vi "MaxEye_ATE_Create Configuration Variable to Text.vi"(0 "Variant":variant, 11 "error in (no error)":errorcluster) -> (4 "concatenated string":string, 15 "error out":errorcluster)   [LabVIEW 2021]
uses:
  <vilib>/Utility/Data Type/NI_Data Type.lvlib
  <userlib>/_OpenG.lib/lvdata/lvdata.llb/openg_variant.lvlib
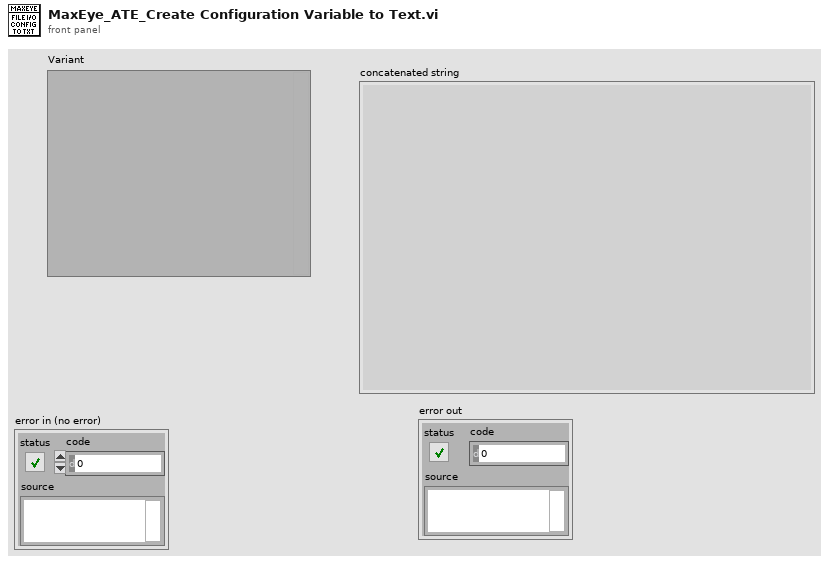
[diagram p1: front panel]
types:
  T1 = typedef "NI_Data Type.lvlib/Data Type.ctl" = enum8{"Invalid Type", "Void", "I8", "I16", "I32", "I64", "U8", "U16", "U32", "U64", "Single Float", "Double Float", "Extended Float", "Single Complex", "Double Complex", "Extended Complex", "Enum U8", "Enum U16", "Enum U32", "Enum U64", "Single Float With Unit", "Double Float With Unit", "Extended Float With Unit", "Single Complex with Unit", "Double Complex with Unit", "Extended Complex with Unit", "Boolean", "String", "Path", "Picture", "Tag", "Array", "Cluster", "Variant", "LV Variant", "Waveform", "Timestamp", "Digital Waveform", "Digital Data", "ExpressData", "Refnum", "External Data", "VI", "Poly VI", "LabVIEW Class Instance", "Fixed Point", "Set Collection", "Map Collection"}
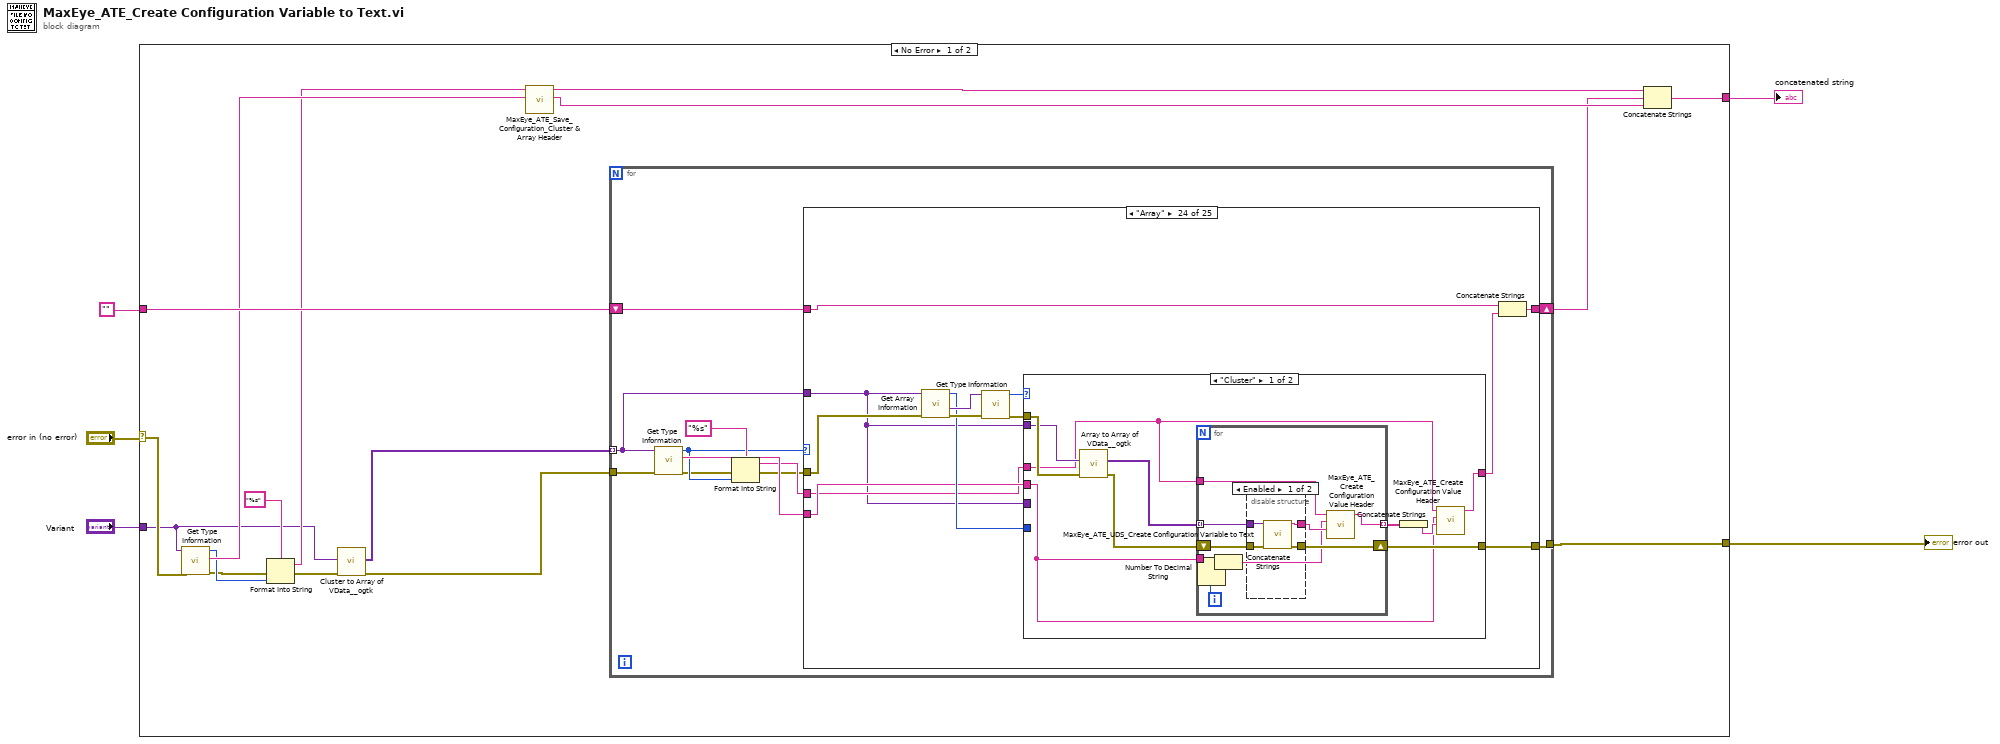
[diagram p0: block diagram]
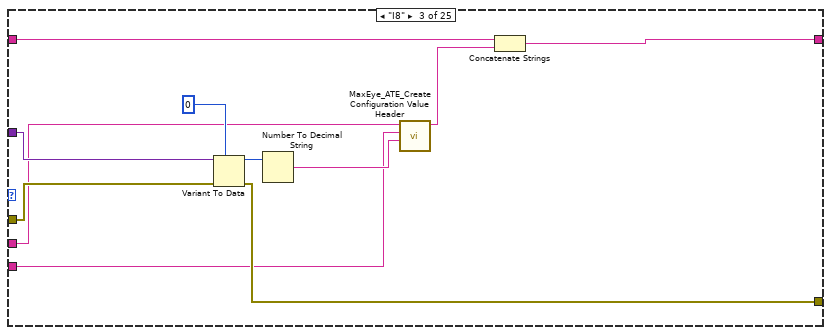
[diagram p4: hidden frame]
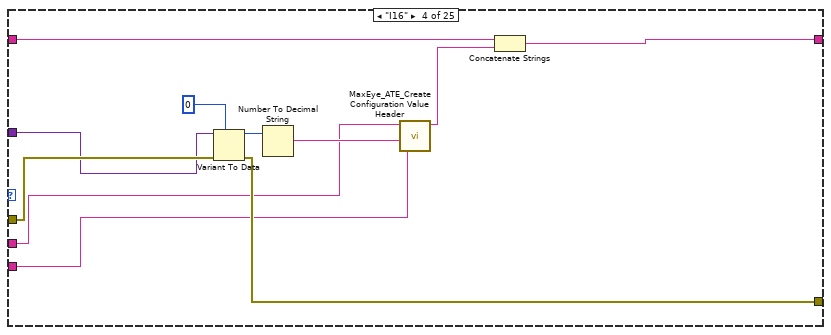
[diagram p5: hidden frame]
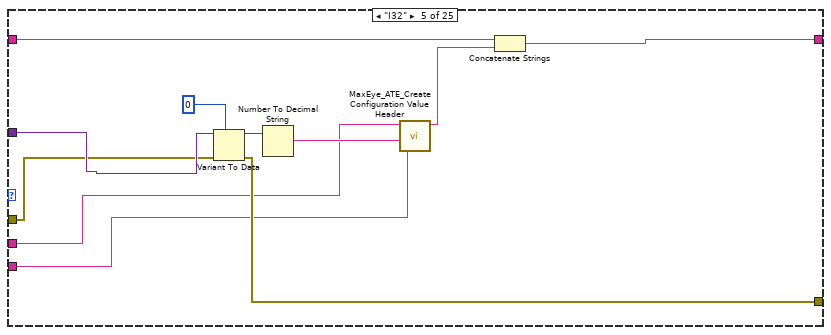
[diagram p6: hidden frame]
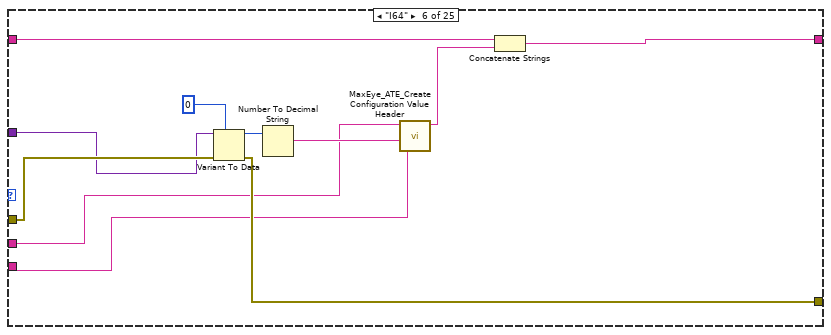
[diagram p7: hidden frame]
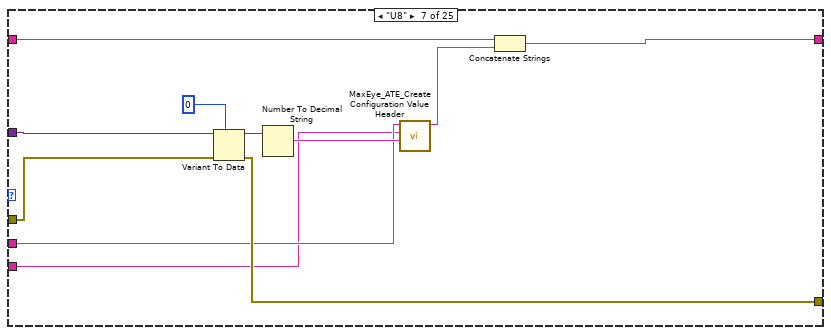
[diagram p8: hidden frame]
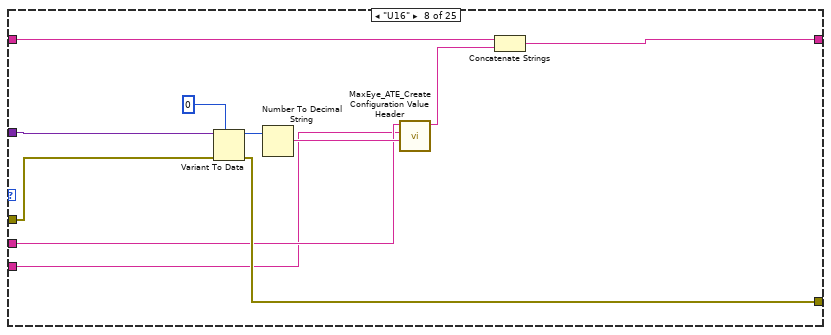
[diagram p9: hidden frame]
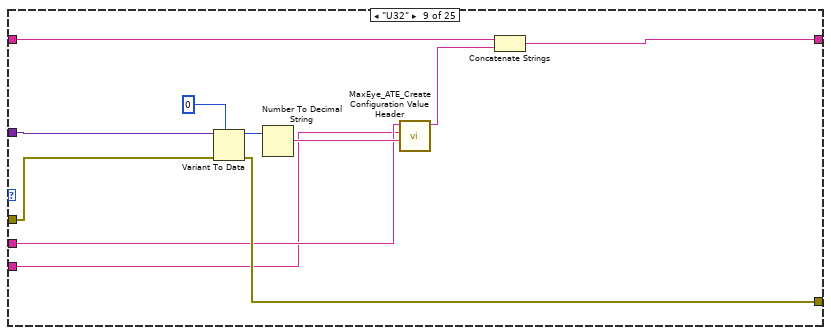
[diagram p10: hidden frame]
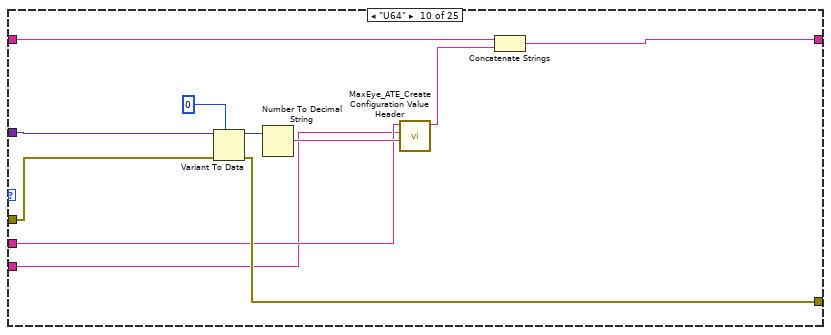
[diagram p11: hidden frame]
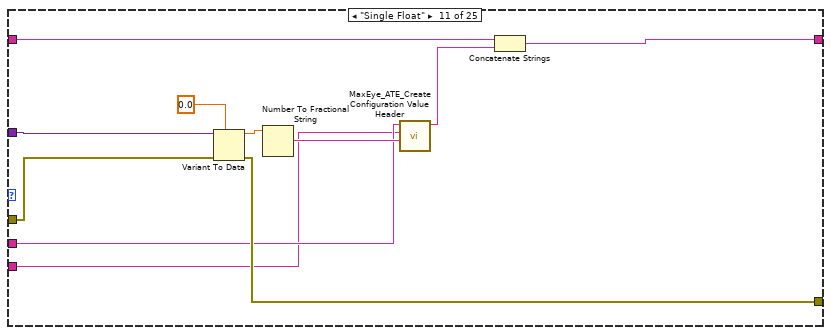
[diagram p12: hidden frame]
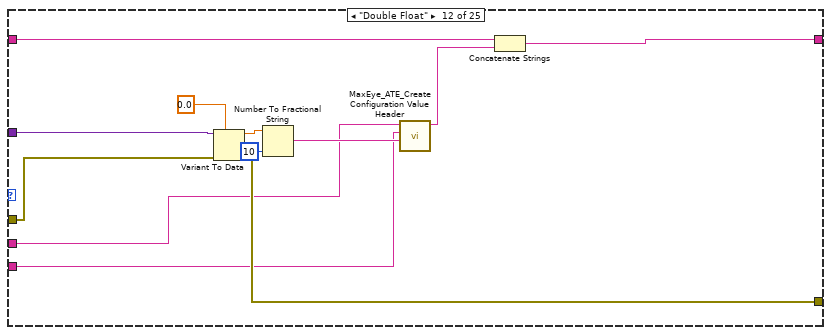
[diagram p13: hidden frame]
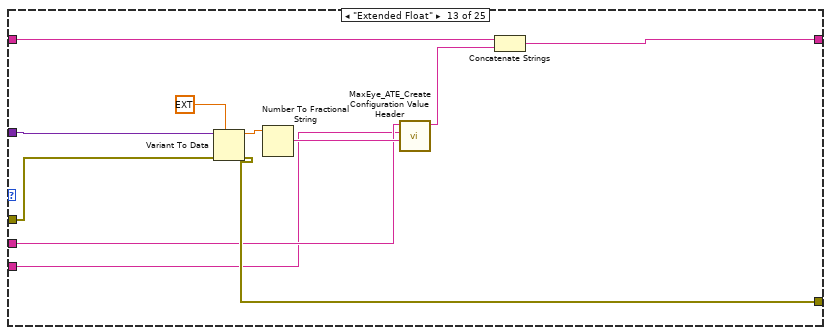
[diagram p14: hidden frame]
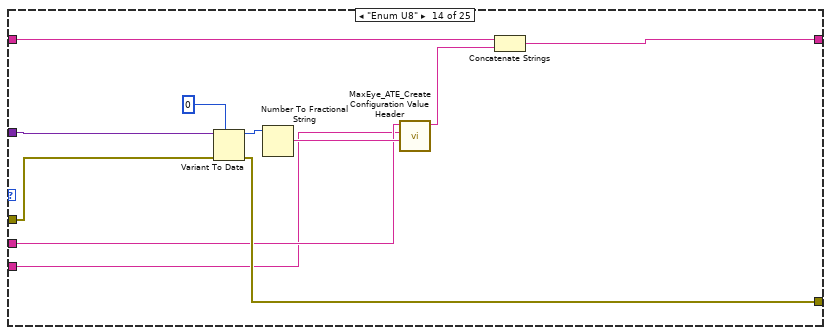
[diagram p15: hidden frame]
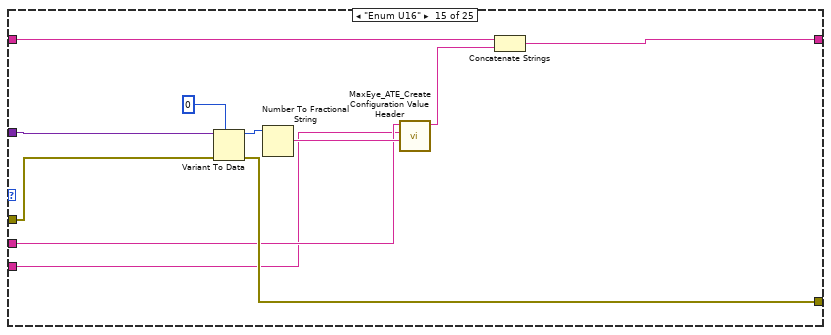
[diagram p16: hidden frame]
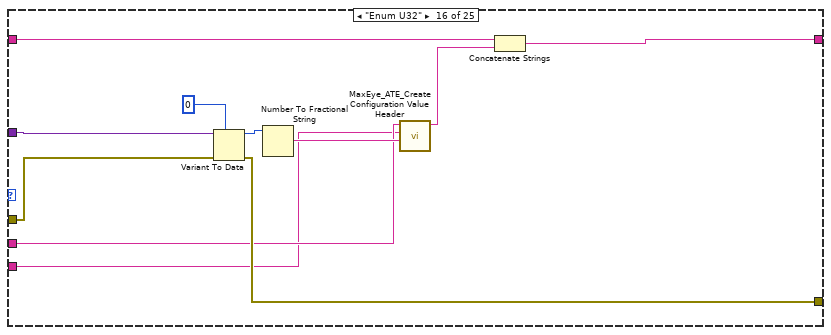
[diagram p17: hidden frame]
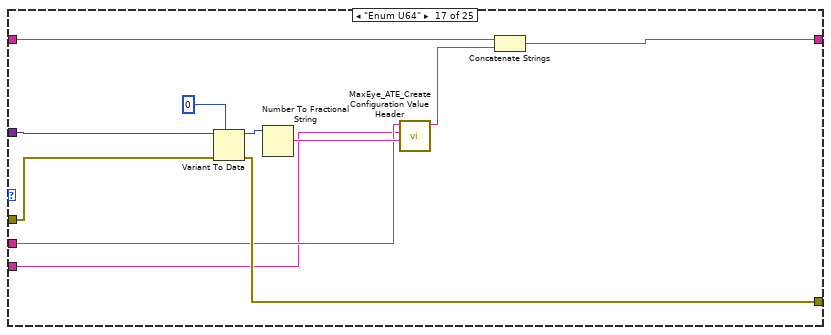
[diagram p18: hidden frame]
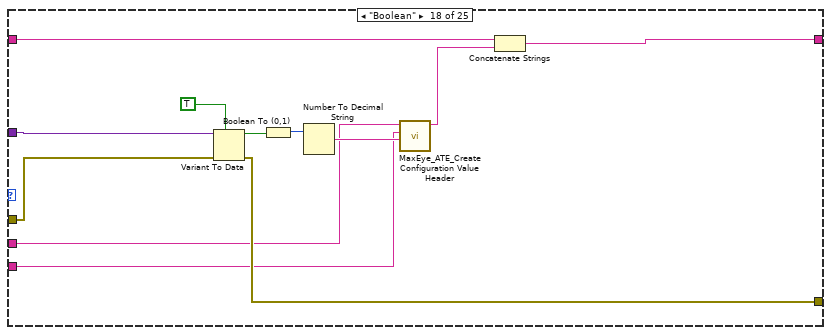
[diagram p19: hidden frame]
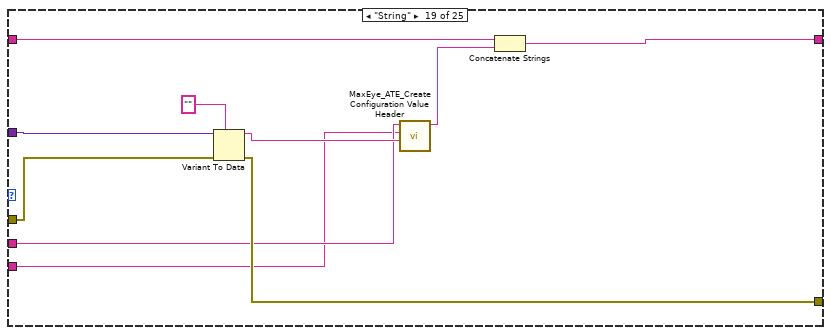
[diagram p20: hidden frame]
diagram:
  n1 = case shown="No Error" "error in (no error)" {
    selector: "error in (no error)" -> [w15 w1033]
    tunnel: "" -> [w21 w1032]
    tunnel: [w17 w1032] -> w4
    tunnel: [w16 w1033] -> w2
    tunnel: "Variant" -> [w9 _]
    frame No Error {
      n2 = call <vilib>:"Get Type Information.vi"("error in (no error)"=w15, "variant"=w9) -> ("error out"=w10:errorcluster, "name"=w14:string, "type"=w13:T1)  [unwired: 5 in, 2 out]
      n3 = Format Into String(format string="%s", error in=w10, w13) -> (resulting string=w11:string, error out=w6:errorcluster)  [unwired: 1 in]
      n4 = call <userlib>:"Cluster to Array of VData__ogtk.vi"("error in (no error)"=w6, "Cluster"=w9) -> ("error out"=w7:errorcluster, "Array of VData"=w8:variant[])  [unwired: 8 in]
      n5 = call "MaxEye_ATE_Save_Configuration_Cluster & Array Header.vi"("Label Name"=w14, "Class Name"=w11) -> ("End"=w19:string, "Begin"=w20:string)  [unwired: 8 in]
      n6 = for {
        tunnel: w7 -> [w32]
        shift-right: [w30] -> w18
        shift-left: w21 -> [w31]
        tunnel: [w29] -> w16
        tunnel: w8 -> [w22] mode=indexing
        n7 = call <vilib>:"Get Type Information.vi"("error in (no error)"=w32, "variant"=w22) -> ("error out"=w23:errorcluster, "name"=w28:string, "type"=w26:T1)  [unwired: 5 in, 2 out]
        n8 = Format Into String(format string="%s", error in=w23, w26) -> (resulting string=w25:string, error out=w24:errorcluster)  [unwired: 1 in]
        n9 = case shown="\"Array\"" w26 {
          tunnel: w24 -> [w33 w35 w47 w51 w61 w73 w91 w102 w113 w124 w135 w147 w158 w169 w180 w191 w202 w214 w224 w235 w244 w247 w264 w277 w1031]
          tunnel: w31 -> [w34 w36 w44 w56 w67 w78 w88 w99 w110 w121 w132 w144 w155 w166 w177 w188 w199 w212 w222 w233 w243 w255 w263 w276 w1030]
          tunnel: [w34 w36 w43 w55 w66 w77 w87 w98 w109 w120 w131 w143 w154 w165 w176 w187 w198 w211 w221 w232 w242 w254 w262 w275 w1029] -> w30
          tunnel: [w33 w35 w40 w52 w63 w74 w84 w95 w106 w117 w128 w140 w151 w162 w173 w184 w195 w206 w218 w228 w244 w247 w264 w268 w1028] -> w29
          tunnel: w28 -> [_ _ w37 w49 w59 w70 w81 w92 w103 w114 w125 w139 w148 w159 w170 w181 w192 w203 w215 w225 w239 w251 w259 w267 _]
          tunnel: w25 -> [_ _ w38 w50 w60 w71 w82 w93 w104 w115 w126 w138 w149 w160 w171 w182 w193 w204 w216 w226 w240 w252 w260 w266 _]
          tunnel: w22 -> [_ _ w39 w48 w62 w72 w83 w94 w105 w116 w127 w137 w150 w161 w172 w183 w194 w205 w217 w227 w238 w250 w258 w265 w1026]
          frame "Invalid Type", Default {
          }
          frame "Void" {
          }
          frame "I8" {
            n10 = Variant To Data(error in=w47, type=i8 0, Variant=w39) -> (data=w45:i8, error out=w40:errorcluster)
            n11 = Number To Decimal String(number=w45) -> (decimal integer string=w42:string)  [unwired: 1 in]
            n12 = call "MaxEye_ATE_Create Configuration Value Header.vi"("Class_value"=w42, "Label_name"=w37, "Class_name"=w38) -> ("Encoded Value"=w41:string)  [unwired: 8 in]
            n13 = Concatenate Strings(w44, w41) -> (w43:string)
          }
          frame "I16" {
            n14 = Variant To Data(error in=w51, type=i16 0, Variant=w48) -> (data=w57:i16, error out=w52:errorcluster)
            n15 = Number To Decimal String(number=w57) -> (decimal integer string=w54:string)  [unwired: 1 in]
            n16 = call "MaxEye_ATE_Create Configuration Value Header.vi"("Class_value"=w54, "Label_name"=w49, "Class_name"=w50) -> ("Encoded Value"=w53:string)  [unwired: 8 in]
            n17 = Concatenate Strings(w56, w53) -> (w55:string)
          }
          frame "I32" {
            n18 = Variant To Data(error in=w61, type=0, Variant=w62) -> (data=w68:i32, error out=w63:errorcluster)
            n19 = Number To Decimal String(number=w68) -> (decimal integer string=w65:string)  [unwired: 1 in]
            n20 = call "MaxEye_ATE_Create Configuration Value Header.vi"("Class_value"=w65, "Label_name"=w59, "Class_name"=w60) -> ("Encoded Value"=w64:string)  [unwired: 8 in]
            n21 = Concatenate Strings(w67, w64) -> (w66:string)
          }
          frame "I64" {
            n22 = Variant To Data(error in=w73, type=i64 0, Variant=w72) -> (data=w79:i64, error out=w74:errorcluster)
            n23 = Number To Decimal String(number=w79) -> (decimal integer string=w76:string)  [unwired: 1 in]
            n24 = call "MaxEye_ATE_Create Configuration Value Header.vi"("Class_value"=w76, "Label_name"=w70, "Class_name"=w71) -> ("Encoded Value"=w75:string)  [unwired: 8 in]
            n25 = Concatenate Strings(w78, w75) -> (w77:string)
          }
          frame "U8" {
            n26 = Variant To Data(error in=w91, type=u8 0, Variant=w83) -> (data=w89:u8, error out=w84:errorcluster)
            n27 = Number To Decimal String(number=w89) -> (decimal integer string=w86:string)  [unwired: 1 in]
            n28 = call "MaxEye_ATE_Create Configuration Value Header.vi"("Class_value"=w86, "Label_name"=w81, "Class_name"=w82) -> ("Encoded Value"=w85:string)  [unwired: 8 in]
            n29 = Concatenate Strings(w88, w85) -> (w87:string)
          }
          frame "U16" {
            n30 = Variant To Data(error in=w102, type=u16 0, Variant=w94) -> (data=w100:u16, error out=w95:errorcluster)
            n31 = Number To Decimal String(number=w100) -> (decimal integer string=w97:string)  [unwired: 1 in]
            n32 = call "MaxEye_ATE_Create Configuration Value Header.vi"("Class_value"=w97, "Label_name"=w92, "Class_name"=w93) -> ("Encoded Value"=w96:string)  [unwired: 8 in]
            n33 = Concatenate Strings(w99, w96) -> (w98:string)
          }
          frame "U32" {
            n34 = Variant To Data(error in=w113, type=u32 0, Variant=w105) -> (data=w111:u32, error out=w106:errorcluster)
            n35 = Number To Decimal String(number=w111) -> (decimal integer string=w108:string)  [unwired: 1 in]
            n36 = call "MaxEye_ATE_Create Configuration Value Header.vi"("Class_value"=w108, "Label_name"=w103, "Class_name"=w104) -> ("Encoded Value"=w107:string)  [unwired: 8 in]
            n37 = Concatenate Strings(w110, w107) -> (w109:string)
          }
          frame "U64" {
            n38 = Variant To Data(error in=w124, type=u64 0, Variant=w116) -> (data=w122:u64, error out=w117:errorcluster)
            n39 = Number To Decimal String(number=w122) -> (decimal integer string=w119:string)  [unwired: 1 in]
            n40 = call "MaxEye_ATE_Create Configuration Value Header.vi"("Class_value"=w119, "Label_name"=w114, "Class_name"=w115) -> ("Encoded Value"=w118:string)  [unwired: 8 in]
            n41 = Concatenate Strings(w121, w118) -> (w120:string)
          }
          frame "Single Float" {
            n42 = Variant To Data(error in=w135, type=sgl 0.0, Variant=w127) -> (data=w133:sgl, error out=w128:errorcluster)
            n43 = Number To Fractional String(number=w133) -> (F-format string=w130:string)  [unwired: 3 in]
            n44 = call "MaxEye_ATE_Create Configuration Value Header.vi"("Class_value"=w130, "Label_name"=w125, "Class_name"=w126) -> ("Encoded Value"=w129:string)  [unwired: 8 in]
            n45 = Concatenate Strings(w132, w129) -> (w131:string)
          }
          frame "Double Float" {
            n46 = Variant To Data(error in=w147, type=0.0, Variant=w137) -> (data=w145:dbl, error out=w140:errorcluster)
            n47 = Number To Fractional String(number=w145, precision (6)=i16 10) -> (F-format string=w142:string)  [unwired: 2 in]
            n48 = call "MaxEye_ATE_Create Configuration Value Header.vi"("Class_value"=w142, "Label_name"=w139, "Class_name"=w138) -> ("Encoded Value"=w141:string)  [unwired: 8 in]
            n49 = Concatenate Strings(w144, w141) -> (w143:string)
          }
          frame "Extended Float" {
            n50 = Variant To Data(error in=w158, type=ext 0.0, Variant=w150) -> (data=w156:ext, error out=w151:errorcluster)
            n51 = Number To Fractional String(number=w156) -> (F-format string=w153:string)  [unwired: 3 in]
            n52 = call "MaxEye_ATE_Create Configuration Value Header.vi"("Class_value"=w153, "Label_name"=w148, "Class_name"=w149) -> ("Encoded Value"=w152:string)  [unwired: 8 in]
            n53 = Concatenate Strings(w155, w152) -> (w154:string)
          }
          frame "Enum U8" {
            n54 = Variant To Data(error in=w169, type=u8 0, Variant=w161) -> (data=w167:u8, error out=w162:errorcluster)
            n55 = Number To Fractional String(number=w167) -> (F-format string=w164:string)  [unwired: 3 in]
            n56 = call "MaxEye_ATE_Create Configuration Value Header.vi"("Class_value"=w164, "Label_name"=w159, "Class_name"=w160) -> ("Encoded Value"=w163:string)  [unwired: 8 in]
            n57 = Concatenate Strings(w166, w163) -> (w165:string)
          }
          frame "Enum U16" {
            n58 = Variant To Data(error in=w180, type=u16 0, Variant=w172) -> (data=w178:u16, error out=w173:errorcluster)
            n59 = Number To Fractional String(number=w178) -> (F-format string=w175:string)  [unwired: 3 in]
            n60 = call "MaxEye_ATE_Create Configuration Value Header.vi"("Class_value"=w175, "Label_name"=w170, "Class_name"=w171) -> ("Encoded Value"=w174:string)  [unwired: 8 in]
            n61 = Concatenate Strings(w177, w174) -> (w176:string)
          }
          frame "Enum U32" {
            n62 = Variant To Data(error in=w191, type=u32 0, Variant=w183) -> (data=w189:u32, error out=w184:errorcluster)
            n63 = Number To Fractional String(number=w189) -> (F-format string=w186:string)  [unwired: 3 in]
            n64 = call "MaxEye_ATE_Create Configuration Value Header.vi"("Class_value"=w186, "Label_name"=w181, "Class_name"=w182) -> ("Encoded Value"=w185:string)  [unwired: 8 in]
            n65 = Concatenate Strings(w188, w185) -> (w187:string)
          }
          frame "Enum U64" {
            n66 = Variant To Data(error in=w202, type=u64 0, Variant=w194) -> (data=w200:u64, error out=w195:errorcluster)
            n67 = Number To Fractional String(number=w200) -> (F-format string=w197:string)  [unwired: 3 in]
            n68 = call "MaxEye_ATE_Create Configuration Value Header.vi"("Class_value"=w197, "Label_name"=w192, "Class_name"=w193) -> ("Encoded Value"=w196:string)  [unwired: 8 in]
            n69 = Concatenate Strings(w199, w196) -> (w198:string)
          }
          frame "Boolean" {
            n70 = Variant To Data(error in=w214, type=TRUE, Variant=w205) -> (data=w209:bool, error out=w206:errorcluster)
            n71 = Boolean To (0,1)(Boolean=w209) -> (0, 1=w208:i16)
            n72 = Number To Decimal String(number=w208) -> (decimal integer string=w207:string)  [unwired: 1 in]
            n73 = call "MaxEye_ATE_Create Configuration Value Header.vi"("Class_value"=w207, "Label_name"=w203, "Class_name"=w204) -> ("Encoded Value"=w210:string)  [unwired: 8 in]
            n74 = Concatenate Strings(w212, w210) -> (w211:string)
          }
          frame "String" {
            n75 = Variant To Data(error in=w224, type="", Variant=w217) -> (data=w219:string, error out=w218:errorcluster)
            n76 = call "MaxEye_ATE_Create Configuration Value Header.vi"("Class_value"=w219, "Label_name"=w215, "Class_name"=w216) -> ("Encoded Value"=w220:string)  [unwired: 8 in]
            n77 = Concatenate Strings(w222, w220) -> (w221:string)
          }
          frame "Path" {
            n78 = Variant To Data(error in=w235, type=path "", Variant=w227) -> (data=w230:path, error out=w228:errorcluster)
            n79 = Path To String(path=w230) -> (string=w229:string)
            n80 = call "MaxEye_ATE_Create Configuration Value Header.vi"("Class_value"=w229, "Label_name"=w225, "Class_name"=w226) -> ("Encoded Value"=w231:string)  [unwired: 8 in]
            n81 = Concatenate Strings(w233, w231) -> (w232:string)
          }
          frame "Refnum" {
            n82 = Variant To Data(type="", Variant=w238) -> (data=w236:string)  [unwired: 1 in, 1 out]
            n83 = call "MaxEye_ATE_Create Configuration Value Header.vi"("Class_value"=w236, "Label_name"=w239, "Class_name"=w240) -> ("Encoded Value"=w241:string)  [unwired: 8 in]
            n84 = Concatenate Strings(w243, w241) -> (w242:string)
          }
          frame "Timestamp" {
            n85 = Variant To Data(error in=w247, type=timestamp(0 s since 1904-01-01), Variant=w250) -> (data=w246:timestamp)  [unwired: 1 out]
            n86 = To Double Precision Float(number=w246) -> (double precision float=w245:dbl)
            n87 = Number To Fractional String(number=w245) -> (F-format string=w248:string)  [unwired: 3 in]
            n88 = call "MaxEye_ATE_Create Configuration Value Header.vi"("Class_value"=w248, "Label_name"=w251, "Class_name"=w252) -> ("Encoded Value"=w253:string)  [unwired: 8 in]
            n89 = Concatenate Strings(w255, w253) -> (w254:string)
          }
          frame "Tag" {
            n90 = Variant To Data(type="", Variant=w258) -> (data=w256:string)  [unwired: 1 in, 1 out]
            n91 = call "MaxEye_ATE_Create Configuration Value Header.vi"("Class_value"=w256, "Label_name"=w259, "Class_name"=w260) -> ("Encoded Value"=w261:string)  [unwired: 8 in]
            n92 = Concatenate Strings(w263, w261) -> (w262:string)
          }
          frame "Array" {
            n93 = call <vilib>:"Get Array Information.vi"("error in (no error)"=w277, "variant"=w265) -> ("error out"=w273:errorcluster, "array element data type"=w274:variant, "number of dimensions"=w272:i32)  [unwired: 6 in, 1 out]
            n94 = call <vilib>:"Get Type Information.vi"("error in (no error)"=w273, "variant"=w274) -> ("error out"=w270:errorcluster, "type"=w271:T1)  [unwired: 5 in, 3 out]
            n95 = case shown="\"Cluster\"" w271 {
              selector: w271 -> [_ w308]
              tunnel: w272 -> [_ w309]
              tunnel: w270 -> [w287 w304]
              tunnel: w266 -> [w279 w307]
              tunnel: w267 -> [w278 w306]
              tunnel: w265 -> [_ w305]
              tunnel: [w281 w303] -> w269
              tunnel: [w283 w302] -> w268
              tunnel: w265 -> [w286 _]
              frame "Cluster" {
                n96 = call <userlib>:"Array to Array of VData__ogtk.vi"("error in (no error)"=w287, "MultiD Array"=w286) -> ("error out"=w284:errorcluster, "1D Array of Variants"=w285:variant[])  [unwired: 8 in]
                n97 = for {
                  tunnel: w285 -> [w297] mode=indexing
                  tunnel: [w293] -> w282 mode=indexing
                  shift-right: [w295] -> w283
                  shift-left: w284 -> [w296]
                  tunnel: w279 -> [w292]
                  tunnel: w278 -> [w291]
                  i -> [w290]
                  n98 = Number To Decimal String(number=w290) -> (decimal integer string=w289:string)  [unwired: 1 in]
                  n99 = Concatenate Strings(w291, w289) -> (w288:string)
                  n100 = disable-structure shown="Enabled" {
                    disable-tunnel: w297 -> [w298 _]
                    disable-tunnel: w296 -> [w301 _]
                    disable-tunnel: [w300 _] -> w295
                    disable-tunnel: [w299 _] -> w294
                    frame Enabled {
                      n101 = call "MaxEye_ATE_UDS_Create Configuration Variable to Text.vi"("Variant"=w298, "error in (no error)"=w301) -> ("concatenated string"=w299:string, "error out"=w300:errorcluster)  [unwired: 12 in]
                    }
                    frame Disabled {
                    }
                  }
                  n102 = call "MaxEye_ATE_Create Configuration Value Header.vi"("Class_value"=w294, "Label_name"=w288, "Class_name"=w292) -> ("Encoded Value"=w293:string)  [unwired: 8 in]
                }
                n103 = Concatenate Strings(w282) -> (w280:string)
                n104 = call "MaxEye_ATE_Create Configuration Value Header.vi"("Class_value"=w280, "Label_name"=w278, "Class_name"=w279) -> ("Encoded Value"=w281:string)  [unwired: 8 in]
              }
              frame "Void", Default {
                n105 = case shown="1" w309 {
                  tunnel: w308 -> [_ w317 w574 w803]
                  tunnel: w307 -> [_ w316 w573 w802]
                  tunnel: w306 -> [_ w315 w572 w801]
                  tunnel: w305 -> [_ w314 w571 w800]
                  tunnel: w304 -> [w310 w313 w570 w799]
                  tunnel: [_ w312 w569 w798] -> w303
                  tunnel: [w310 w311 w568 w797] -> w302
                  frame 0, Default {
                  }
                  frame 1 {
                    n106 = case shown="\"Enum U32\"" w317 {
                      tunnel: w316 -> [w328 w339 w350 w361 w372 w383 w394 w405 w416 w427 w438 w449 w460 w473 w484 w495 w506 w517 w528 w539 w551 w566 _]
                      tunnel: w315 -> [w327 w338 w349 w360 w371 w382 w393 w404 w415 w426 w437 w448 w459 w472 w483 w494 w505 w516 w527 w538 w550 w565 _]
                      tunnel: w314 -> [w325 w336 w347 w358 w369 w380 w391 w402 w413 w424 w435 w446 w457 w464 w481 w492 w503 w514 w525 w536 w548 w563 _]
                      tunnel: w313 -> [w326 w337 w348 w359 w370 w381 w392 w403 w414 w425 w436 w447 w458 w463 w482 w493 w504 w515 w526 w537 w549 w564 w567]
                      tunnel: [w319 w330 w341 w352 w363 w374 w385 w396 w407 w418 w429 w440 w451 w468 w475 w486 w497 w508 w519 w530 w543 w557 _] -> w312
                      tunnel: [w318 w329 w340 w351 w362 w373 w384 w395 w406 w417 w428 w439 w450 w462 w474 w485 w496 w507 w518 w529 w542 w555 w567] -> w311
                      frame "I8" {
                        n107 = Variant To Data(error in=w326, type=i8[] [], Variant=w325) -> (data=w323:i8[], error out=w318:errorcluster)
                        n108 = Array To Spreadsheet String(delimiter (Tab)=",", array=w323, 3:"%s" ("format string")) -> (spreadsheet string=w320:string)
                        n109 = call "MaxEye_ATE_Create Configuration Value Header.vi"("Class_value"=w320, "Label_name"=w327, "Class_name"=w328) -> ("Encoded Value"=w319:string)  [unwired: 8 in]
                      }
                      frame "I16" {
                        n110 = Variant To Data(error in=w337, type=i16[] [], Variant=w336) -> (data=w334:i16[], error out=w329:errorcluster)
                        n111 = Array To Spreadsheet String(delimiter (Tab)=",", array=w334, 3:"%s" ("format string")) -> (spreadsheet string=w331:string)
                        n112 = call "MaxEye_ATE_Create Configuration Value Header.vi"("Class_value"=w331, "Label_name"=w338, "Class_name"=w339) -> ("Encoded Value"=w330:string)  [unwired: 8 in]
                      }
                      frame "I32" {
                        n113 = Variant To Data(error in=w348, type=i32[] [], Variant=w347) -> (data=w345:i32[], error out=w340:errorcluster)
                        n114 = Array To Spreadsheet String(delimiter (Tab)=",", array=w345, 3:"%s" ("format string")) -> (spreadsheet string=w342:string)
                        n115 = call "MaxEye_ATE_Create Configuration Value Header.vi"("Class_value"=w342, "Label_name"=w349, "Class_name"=w350) -> ("Encoded Value"=w341:string)  [unwired: 8 in]
                      }
                      frame "I64" {
                        n116 = Variant To Data(error in=w359, type=i64[] [], Variant=w358) -> (data=w356:i64[], error out=w351:errorcluster)
                        n117 = Array To Spreadsheet String(delimiter (Tab)=",", array=w356, 3:"%s" ("format string")) -> (spreadsheet string=w353:string)
                        n118 = call "MaxEye_ATE_Create Configuration Value Header.vi"("Class_value"=w353, "Label_name"=w360, "Class_name"=w361) -> ("Encoded Value"=w352:string)  [unwired: 8 in]
                      }
                      frame "U8" {
                        n119 = Variant To Data(error in=w370, type=u8[] [], Variant=w369) -> (data=w367:u8[], error out=w362:errorcluster)
                        n120 = Array To Spreadsheet String(delimiter (Tab)=",", array=w367, 3:"%s" ("format string")) -> (spreadsheet string=w364:string)
                        n121 = call "MaxEye_ATE_Create Configuration Value Header.vi"("Class_value"=w364, "Label_name"=w371, "Class_name"=w372) -> ("Encoded Value"=w363:string)  [unwired: 8 in]
                      }
                      frame "U16" {
                        n122 = Variant To Data(error in=w381, type=u16[] [], Variant=w380) -> (data=w378:u16[], error out=w373:errorcluster)
                        n123 = Array To Spreadsheet String(delimiter (Tab)=",", array=w378, 3:"%s" ("format string")) -> (spreadsheet string=w375:string)
                        n124 = call "MaxEye_ATE_Create Configuration Value Header.vi"("Class_value"=w375, "Label_name"=w382, "Class_name"=w383) -> ("Encoded Value"=w374:string)  [unwired: 8 in]
                      }
                      frame "U32" {
                        n125 = Variant To Data(error in=w392, type=u32[] [], Variant=w391) -> (data=w389:u32[], error out=w384:errorcluster)
                        n126 = Array To Spreadsheet String(delimiter (Tab)=",", array=w389, 3:"%s" ("format string")) -> (spreadsheet string=w386:string)
                        n127 = call "MaxEye_ATE_Create Configuration Value Header.vi"("Class_value"=w386, "Label_name"=w393, "Class_name"=w394) -> ("Encoded Value"=w385:string)  [unwired: 8 in]
                      }
                      frame "U64" {
                        n128 = Variant To Data(error in=w403, type=u64[] [], Variant=w402) -> (data=w400:u64[], error out=w395:errorcluster)
                        n129 = Array To Spreadsheet String(delimiter (Tab)=",", array=w400, 3:"%s" ("format string")) -> (spreadsheet string=w397:string)
                        n130 = call "MaxEye_ATE_Create Configuration Value Header.vi"("Class_value"=w397, "Label_name"=w404, "Class_name"=w405) -> ("Encoded Value"=w396:string)  [unwired: 8 in]
                      }
                      frame "Single Float" {
                        n131 = Variant To Data(error in=w414, type=sgl[] [], Variant=w413) -> (data=w411:sgl[], error out=w406:errorcluster)
                        n132 = Array To Spreadsheet String(delimiter (Tab)=",", array=w411, 3:"%s" ("format string")) -> (spreadsheet string=w408:string)
                        n133 = call "MaxEye_ATE_Create Configuration Value Header.vi"("Class_value"=w408, "Label_name"=w415, "Class_name"=w416) -> ("Encoded Value"=w407:string)  [unwired: 8 in]
                      }
                      frame "Double Float" {
                        n134 = Variant To Data(error in=w425, type=dbl[] [], Variant=w424) -> (data=w422:dbl[], error out=w417:errorcluster)
                        n135 = Array To Spreadsheet String(delimiter (Tab)=",", array=w422, 3:"%s" ("format string")) -> (spreadsheet string=w419:string)
                        n136 = call "MaxEye_ATE_Create Configuration Value Header.vi"("Class_value"=w419, "Label_name"=w426, "Class_name"=w427) -> ("Encoded Value"=w418:string)  [unwired: 8 in]
                      }
                      frame "Extended Float" {
                        n137 = Variant To Data(error in=w436, type=ext[] [], Variant=w435) -> (data=w433:ext[], error out=w428:errorcluster)
                        n138 = Array To Spreadsheet String(delimiter (Tab)=",", array=w433, 3:"%s" ("format string")) -> (spreadsheet string=w430:string)
                        n139 = call "MaxEye_ATE_Create Configuration Value Header.vi"("Class_value"=w430, "Label_name"=w437, "Class_name"=w438) -> ("Encoded Value"=w429:string)  [unwired: 8 in]
                      }
                      frame "Single Complex" {
                        n140 = Variant To Data(error in=w447, type=ext[] [], Variant=w446) -> (data=w444:ext[], error out=w439:errorcluster)
                        n141 = Array To Spreadsheet String(delimiter (Tab)=",", array=w444, 3:"%s" ("format string")) -> (spreadsheet string=w441:string)
                        n142 = call "MaxEye_ATE_Create Configuration Value Header.vi"("Class_value"=w441, "Label_name"=w448, "Class_name"=w449) -> ("Encoded Value"=w440:string)  [unwired: 8 in]
                      }
                      frame "Double Complex" {
                        n143 = Variant To Data(error in=w458, type=ext[] [], Variant=w457) -> (data=w455:ext[], error out=w450:errorcluster)
                        n144 = Array To Spreadsheet String(delimiter (Tab)=",", array=w455, 3:"%s" ("format string")) -> (spreadsheet string=w452:string)
                        n145 = call "MaxEye_ATE_Create Configuration Value Header.vi"("Class_value"=w452, "Label_name"=w459, "Class_name"=w460) -> ("Encoded Value"=w451:string)  [unwired: 8 in]
                      }
                      frame "Timestamp" {
                        n146 = Variant To Data(error in=w463, type=timestamp[] [], Variant=w464) -> (data=w466:timestamp[], error out=w462:errorcluster)
                        n147 = To Double Precision Float(number=w466) -> (double precision float=w467:dbl[])
                        n148 = Number To Fractional String(number=w467) -> (F-format string=w461:string[])  [unwired: 3 in]
                        n149 = Array To Spreadsheet String(delimiter (Tab)=",", array=w461, 3:"%s" ("format string")) -> (spreadsheet string=w469:string)
                        n150 = call "MaxEye_ATE_Create Configuration Value Header.vi"("Class_value"=w469, "Label_name"=w472, "Class_name"=w473) -> ("Encoded Value"=w468:string)  [unwired: 8 in]
                      }
                      frame "Extended Complex" {
                        n151 = Variant To Data(error in=w482, type=ext[] [], Variant=w481) -> (data=w479:ext[], error out=w474:errorcluster)
                        n152 = Array To Spreadsheet String(delimiter (Tab)=",", array=w479, 3:"%s" ("format string")) -> (spreadsheet string=w476:string)
                        n153 = call "MaxEye_ATE_Create Configuration Value Header.vi"("Class_value"=w476, "Label_name"=w483, "Class_name"=w484) -> ("Encoded Value"=w475:string)  [unwired: 8 in]
                      }
                      frame "Enum U8" {
                        n154 = Variant To Data(error in=w493, type=u8[] [], Variant=w492) -> (data=w490:u8[], error out=w485:errorcluster)
                        n155 = Array To Spreadsheet String(delimiter (Tab)=",", array=w490, 3:"%s" ("format string")) -> (spreadsheet string=w487:string)
                        n156 = call "MaxEye_ATE_Create Configuration Value Header.vi"("Class_value"=w487, "Label_name"=w494, "Class_name"=w495) -> ("Encoded Value"=w486:string)  [unwired: 8 in]
                      }
                      frame "Enum U16" {
                        n157 = Variant To Data(error in=w504, type=u16[] [], Variant=w503) -> (data=w501:u16[], error out=w496:errorcluster)
                        n158 = Array To Spreadsheet String(delimiter (Tab)=",", array=w501, 3:"%s" ("format string")) -> (spreadsheet string=w498:string)
                        n159 = call "MaxEye_ATE_Create Configuration Value Header.vi"("Class_value"=w498, "Label_name"=w505, "Class_name"=w506) -> ("Encoded Value"=w497:string)  [unwired: 8 in]
                      }
                      frame "Enum U32" {
                        n160 = Variant To Data(error in=w515, type=u32[] [], Variant=w514) -> (data=w512:u32[], error out=w507:errorcluster)
                        n161 = Array To Spreadsheet String(delimiter (Tab)=",", array=w512, 3:"%s" ("format string")) -> (spreadsheet string=w509:string)
                        n162 = call "MaxEye_ATE_Create Configuration Value Header.vi"("Class_value"=w509, "Label_name"=w516, "Class_name"=w517) -> ("Encoded Value"=w508:string)  [unwired: 8 in]
                      }
                      frame "Enum U64" {
                        n163 = Variant To Data(error in=w526, type=u64[] [], Variant=w525) -> (data=w523:u64[], error out=w518:errorcluster)
                        n164 = Array To Spreadsheet String(delimiter (Tab)=",", array=w523, 3:"%s" ("format string")) -> (spreadsheet string=w520:string)
                        n165 = call "MaxEye_ATE_Create Configuration Value Header.vi"("Class_value"=w520, "Label_name"=w527, "Class_name"=w528) -> ("Encoded Value"=w519:string)  [unwired: 8 in]
                      }
                      frame "String" {
                        n166 = Variant To Data(error in=w537, type=string[] [], Variant=w536) -> (data=w534:string[], error out=w529:errorcluster)
                        n167 = Array To Spreadsheet String(delimiter (Tab)=",", array=w534, 3:"%s" ("format string")) -> (spreadsheet string=w531:string)
                        n168 = call "MaxEye_ATE_Create Configuration Value Header.vi"("Class_value"=w531, "Label_name"=w538, "Class_name"=w539) -> ("Encoded Value"=w530:string)  [unwired: 8 in]
                      }
                      frame "Refnum" {
                        n169 = Variant To Data(error in=w549, type=refnum<k21>[] [""], Variant=w548) -> (data=w541:refnum<k21>[], error out=w542:errorcluster)
                        n170 = for {
                          tunnel: w541 -> [w553] mode=indexing
                          tunnel: [w554] -> w540 mode=indexing
                          n171 = Variant To Data(type="", Variant=w553) -> (data=w554:string)  [unwired: 1 in, 1 out]
                        }
                        n172 = Array To Spreadsheet String(delimiter (Tab)=",", array=w540, 3:"%s" ("format string")) -> (spreadsheet string=w544:string)
                        n173 = call "MaxEye_ATE_Create Configuration Value Header.vi"("Class_value"=w544, "Label_name"=w550, "Class_name"=w551) -> ("Encoded Value"=w543:string)  [unwired: 8 in]
                      }
                      frame "Boolean" {
                        n174 = Variant To Data(error in=w564, type=bool[] [], Variant=w563) -> (data=w561:bool[], error out=w555:errorcluster)
                        n175 = Boolean To (0,1)(Boolean=w561) -> (0, 1=w556:i16[])
                        n176 = Array To Spreadsheet String(delimiter (Tab)=",", array=w556, 3:"%s" ("format string")) -> (spreadsheet string=w558:string)
                        n177 = call "MaxEye_ATE_Create Configuration Value Header.vi"("Class_value"=w558, "Label_name"=w565, "Class_name"=w566) -> ("Encoded Value"=w557:string)  [unwired: 8 in]
                      }
                      frame "Void", Default {
                      }
                    }
                  }
                  frame 2 {
                    n178 = case shown="\"Double Complex\"" w574 {
                      tunnel: w573 -> [w585 w596 w607 w618 w629 w640 w651 w662 w673 w684 w695 w706 w717 w728 w739 w750 w761 w772 w783 w795 _]
                      tunnel: w572 -> [w584 w595 w606 w617 w628 w639 w650 w661 w672 w683 w694 w705 w716 w727 w738 w749 w760 w771 w782 w794 _]
                      tunnel: w571 -> [w582 w593 w604 w615 w626 w637 w648 w659 w670 w681 w692 w703 w714 w725 w736 w747 w758 w769 w780 w792 _]
                      tunnel: w570 -> [w583 w594 w605 w616 w627 w638 w649 w660 w671 w682 w693 w704 w715 w726 w737 w748 w759 w770 w781 w793 w796]
                      tunnel: [w576 w587 w598 w609 w620 w631 w642 w653 w664 w675 w686 w697 w708 w719 w730 w741 w752 w763 w774 w786 _] -> w569
                      tunnel: [w575 w586 w597 w608 w619 w630 w641 w652 w663 w674 w685 w696 w707 w718 w729 w740 w751 w762 w773 w784 w796] -> w568
                      frame "I8" {
                        n179 = Variant To Data(error in=w583, type=i8[][] [], Variant=w582) -> (data=w580:i8[][], error out=w575:errorcluster)
                        n180 = Array To Spreadsheet String(delimiter (Tab)=",", array=w580, 3:"%s" ("format string")) -> (spreadsheet string=w577:string)
                        n181 = call "MaxEye_ATE_Create Configuration Value Header.vi"("Class_value"=w577, "Label_name"=w584, "Class_name"=w585) -> ("Encoded Value"=w576:string)  [unwired: 8 in]
                      }
                      frame "I16" {
                        n182 = Variant To Data(error in=w594, type=i16[][] [], Variant=w593) -> (data=w591:i16[][], error out=w586:errorcluster)
                        n183 = Array To Spreadsheet String(delimiter (Tab)=",", array=w591, 3:"%s" ("format string")) -> (spreadsheet string=w588:string)
                        n184 = call "MaxEye_ATE_Create Configuration Value Header.vi"("Class_value"=w588, "Label_name"=w595, "Class_name"=w596) -> ("Encoded Value"=w587:string)  [unwired: 8 in]
                      }
                      frame "I32" {
                        n185 = Variant To Data(error in=w605, type=i32[][] [], Variant=w604) -> (data=w602:i32[][], error out=w597:errorcluster)
                        n186 = Array To Spreadsheet String(delimiter (Tab)=",", array=w602, 3:"%s" ("format string")) -> (spreadsheet string=w599:string)
                        n187 = call "MaxEye_ATE_Create Configuration Value Header.vi"("Class_value"=w599, "Label_name"=w606, "Class_name"=w607) -> ("Encoded Value"=w598:string)  [unwired: 8 in]
                      }
                      frame "I64" {
                        n188 = Variant To Data(error in=w616, type=i64[][] [], Variant=w615) -> (data=w613:i64[][], error out=w608:errorcluster)
                        n189 = Array To Spreadsheet String(delimiter (Tab)=",", array=w613, 3:"%s" ("format string")) -> (spreadsheet string=w610:string)
                        n190 = call "MaxEye_ATE_Create Configuration Value Header.vi"("Class_value"=w610, "Label_name"=w617, "Class_name"=w618) -> ("Encoded Value"=w609:string)  [unwired: 8 in]
                      }
                      frame "U8" {
                        n191 = Variant To Data(error in=w627, type=u8[][] [], Variant=w626) -> (data=w624:u8[][], error out=w619:errorcluster)
                        n192 = Array To Spreadsheet String(delimiter (Tab)=",", array=w624, 3:"%s" ("format string")) -> (spreadsheet string=w621:string)
                        n193 = call "MaxEye_ATE_Create Configuration Value Header.vi"("Class_value"=w621, "Label_name"=w628, "Class_name"=w629) -> ("Encoded Value"=w620:string)  [unwired: 8 in]
                      }
                      frame "U16" {
                        n194 = Variant To Data(error in=w638, type=u16[][] [], Variant=w637) -> (data=w635:u16[][], error out=w630:errorcluster)
                        n195 = Array To Spreadsheet String(delimiter (Tab)=",", array=w635, 3:"%s" ("format string")) -> (spreadsheet string=w632:string)
                        n196 = call "MaxEye_ATE_Create Configuration Value Header.vi"("Class_value"=w632, "Label_name"=w639, "Class_name"=w640) -> ("Encoded Value"=w631:string)  [unwired: 8 in]
                      }
                      frame "U32" {
                        n197 = Variant To Data(error in=w649, type=u32[][] [], Variant=w648) -> (data=w646:u32[][], error out=w641:errorcluster)
                        n198 = Array To Spreadsheet String(delimiter (Tab)=",", array=w646, 3:"%s" ("format string")) -> (spreadsheet string=w643:string)
                        n199 = call "MaxEye_ATE_Create Configuration Value Header.vi"("Class_value"=w643, "Label_name"=w650, "Class_name"=w651) -> ("Encoded Value"=w642:string)  [unwired: 8 in]
                      }
                      frame "U64" {
                        n200 = Variant To Data(error in=w660, type=u64[][] [], Variant=w659) -> (data=w657:u64[][], error out=w652:errorcluster)
                        n201 = Array To Spreadsheet String(delimiter (Tab)=",", array=w657, 3:"%s" ("format string")) -> (spreadsheet string=w654:string)
                        n202 = call "MaxEye_ATE_Create Configuration Value Header.vi"("Class_value"=w654, "Label_name"=w661, "Class_name"=w662) -> ("Encoded Value"=w653:string)  [unwired: 8 in]
                      }
                      frame "Single Float" {
                        n203 = Variant To Data(error in=w671, type=sgl[][] [], Variant=w670) -> (data=w668:sgl[][], error out=w663:errorcluster)
                        n204 = Array To Spreadsheet String(delimiter (Tab)=",", array=w668, 3:"%s" ("format string")) -> (spreadsheet string=w665:string)
                        n205 = call "MaxEye_ATE_Create Configuration Value Header.vi"("Class_value"=w665, "Label_name"=w672, "Class_name"=w673) -> ("Encoded Value"=w664:string)  [unwired: 8 in]
                      }
                      frame "Double Float" {
                        n206 = Variant To Data(error in=w682, type=dbl[][] [], Variant=w681) -> (data=w679:dbl[][], error out=w674:errorcluster)
                        n207 = Array To Spreadsheet String(delimiter (Tab)=",", array=w679, 3:"%s" ("format string")) -> (spreadsheet string=w676:string)
                        n208 = call "MaxEye_ATE_Create Configuration Value Header.vi"("Class_value"=w676, "Label_name"=w683, "Class_name"=w684) -> ("Encoded Value"=w675:string)  [unwired: 8 in]
                      }
                      frame "Extended Float" {
                        n209 = Variant To Data(error in=w693, type=ext[][] [], Variant=w692) -> (data=w690:ext[][], error out=w685:errorcluster)
                        n210 = Array To Spreadsheet String(delimiter (Tab)=",", array=w690, 3:"%s" ("format string")) -> (spreadsheet string=w687:string)
                        n211 = call "MaxEye_ATE_Create Configuration Value Header.vi"("Class_value"=w687, "Label_name"=w694, "Class_name"=w695) -> ("Encoded Value"=w686:string)  [unwired: 8 in]
                      }
                      frame "Single Complex" {
                        n212 = Variant To Data(error in=w704, type=ext[][] [], Variant=w703) -> (data=w701:ext[][], error out=w696:errorcluster)
                        n213 = Array To Spreadsheet String(delimiter (Tab)=",", array=w701, 3:"%s" ("format string")) -> (spreadsheet string=w698:string)
                        n214 = call "MaxEye_ATE_Create Configuration Value Header.vi"("Class_value"=w698, "Label_name"=w705, "Class_name"=w706) -> ("Encoded Value"=w697:string)  [unwired: 8 in]
                      }
                      frame "Double Complex" {
                        n215 = Variant To Data(error in=w715, type=ext[][] [], Variant=w714) -> (data=w712:ext[][], error out=w707:errorcluster)
                        n216 = Array To Spreadsheet String(delimiter (Tab)=",", array=w712, 3:"%s" ("format string")) -> (spreadsheet string=w709:string)
                        n217 = call "MaxEye_ATE_Create Configuration Value Header.vi"("Class_value"=w709, "Label_name"=w716, "Class_name"=w717) -> ("Encoded Value"=w708:string)  [unwired: 8 in]
                      }
                      frame "Extended Complex" {
                        n218 = Variant To Data(error in=w726, type=ext[][] [], Variant=w725) -> (data=w723:ext[][], error out=w718:errorcluster)
                        n219 = Array To Spreadsheet String(delimiter (Tab)=",", array=w723, 3:"%s" ("format string")) -> (spreadsheet string=w720:string)
                        n220 = call "MaxEye_ATE_Create Configuration Value Header.vi"("Class_value"=w720, "Label_name"=w727, "Class_name"=w728) -> ("Encoded Value"=w719:string)  [unwired: 8 in]
                      }
                      frame "Enum U8" {
                        n221 = Variant To Data(error in=w737, type=u8[][] [], Variant=w736) -> (data=w734:u8[][], error out=w729:errorcluster)
                        n222 = Array To Spreadsheet String(delimiter (Tab)=",", array=w734, 3:"%s" ("format string")) -> (spreadsheet string=w731:string)
                        n223 = call "MaxEye_ATE_Create Configuration Value Header.vi"("Class_value"=w731, "Label_name"=w738, "Class_name"=w739) -> ("Encoded Value"=w730:string)  [unwired: 8 in]
                      }
                      frame "Enum U16" {
                        n224 = Variant To Data(error in=w748, type=u16[][] [], Variant=w747) -> (data=w745:u16[][], error out=w740:errorcluster)
                        n225 = Array To Spreadsheet String(delimiter (Tab)=",", array=w745, 3:"%s" ("format string")) -> (spreadsheet string=w742:string)
                        n226 = call "MaxEye_ATE_Create Configuration Value Header.vi"("Class_value"=w742, "Label_name"=w749, "Class_name"=w750) -> ("Encoded Value"=w741:string)  [unwired: 8 in]
                      }
                      frame "Enum U32" {
                        n227 = Variant To Data(error in=w759, type=u32[][] [], Variant=w758) -> (data=w756:u32[][], error out=w751:errorcluster)
                        n228 = Array To Spreadsheet String(delimiter (Tab)=",", array=w756, 3:"%s" ("format string")) -> (spreadsheet string=w753:string)
                        n229 = call "MaxEye_ATE_Create Configuration Value Header.vi"("Class_value"=w753, "Label_name"=w760, "Class_name"=w761) -> ("Encoded Value"=w752:string)  [unwired: 8 in]
                      }
                      frame "Enum U64" {
                        n230 = Variant To Data(error in=w770, type=u64[][] [], Variant=w769) -> (data=w767:u64[][], error out=w762:errorcluster)
                        n231 = Array To Spreadsheet String(delimiter (Tab)=",", array=w767, 3:"%s" ("format string")) -> (spreadsheet string=w764:string)
                        n232 = call "MaxEye_ATE_Create Configuration Value Header.vi"("Class_value"=w764, "Label_name"=w771, "Class_name"=w772) -> ("Encoded Value"=w763:string)  [unwired: 8 in]
                      }
                      frame "String" {
                        n233 = Variant To Data(error in=w781, type=string[][] [], Variant=w780) -> (data=w778:string[][], error out=w773:errorcluster)
                        n234 = Array To Spreadsheet String(delimiter (Tab)=",", array=w778, 3:"%s" ("format string")) -> (spreadsheet string=w775:string)
                        n235 = call "MaxEye_ATE_Create Configuration Value Header.vi"("Class_value"=w775, "Label_name"=w782, "Class_name"=w783) -> ("Encoded Value"=w774:string)  [unwired: 8 in]
                      }
                      frame "Boolean" {
                        n236 = Variant To Data(error in=w793, type=bool[][] [], Variant=w792) -> (data=w790:bool[][], error out=w784:errorcluster)
                        n237 = Boolean To (0,1)(Boolean=w790) -> (0, 1=w785:i16[][])
                        n238 = Array To Spreadsheet String(delimiter (Tab)=",", array=w785, 3:"%s" ("format string")) -> (spreadsheet string=w787:string)
                        n239 = call "MaxEye_ATE_Create Configuration Value Header.vi"("Class_value"=w787, "Label_name"=w794, "Class_name"=w795) -> ("Encoded Value"=w786:string)  [unwired: 8 in]
                      }
                      frame "Void", Default {
                      }
                    }
                  }
                  frame 3 {
                    n240 = case shown="\"Double Complex\"" w803 {
                      tunnel: w802 -> [w814 w825 w836 w847 w858 w869 w880 w891 w902 w913 w924 w935 w946 w957 w968 w979 w990 w1001 w1012 w1024 _]
                      tunnel: w801 -> [w813 w824 w835 w846 w857 w868 w879 w890 w901 w912 w923 w934 w945 w956 w967 w978 w989 w1000 w1011 w1023 _]
                      tunnel: w800 -> [w811 w822 w833 w844 w855 w866 w877 w888 w899 w910 w921 w932 w943 w954 w965 w976 w987 w998 w1009 w1021 _]
                      tunnel: w799 -> [w812 w823 w834 w845 w856 w867 w878 w889 w900 w911 w922 w933 w944 w955 w966 w977 w988 w999 w1010 w1022 w1025]
                      tunnel: [w805 w816 w827 w838 w849 w860 w871 w882 w893 w904 w915 w926 w937 w948 w959 w970 w981 w992 w1003 w1015 _] -> w798
                      tunnel: [w804 w815 w826 w837 w848 w859 w870 w881 w892 w903 w914 w925 w936 w947 w958 w969 w980 w991 w1002 w1013 w1025] -> w797
                      frame "I8" {
                        n241 = Variant To Data(error in=w812, type=i8[][][] [], Variant=w811) -> (data=w809:i8[][][], error out=w804:errorcluster)
                        n242 = Array To Spreadsheet String(delimiter (Tab)=",", array=w809, 3:"%s" ("format string")) -> (spreadsheet string=w806:string)
                        n243 = call "MaxEye_ATE_Create Configuration Value Header.vi"("Class_value"=w806, "Label_name"=w813, "Class_name"=w814) -> ("Encoded Value"=w805:string)  [unwired: 8 in]
                      }
                      frame "I16" {
                        n244 = Variant To Data(error in=w823, type=i16[][][] [], Variant=w822) -> (data=w820:i16[][][], error out=w815:errorcluster)
                        n245 = Array To Spreadsheet String(delimiter (Tab)=",", array=w820, 3:"%s" ("format string")) -> (spreadsheet string=w817:string)
                        n246 = call "MaxEye_ATE_Create Configuration Value Header.vi"("Class_value"=w817, "Label_name"=w824, "Class_name"=w825) -> ("Encoded Value"=w816:string)  [unwired: 8 in]
                      }
                      frame "I32" {
                        n247 = Variant To Data(error in=w834, type=i32[][][] [], Variant=w833) -> (data=w831:i32[][][], error out=w826:errorcluster)
                        n248 = Array To Spreadsheet String(delimiter (Tab)=",", array=w831, 3:"%s" ("format string")) -> (spreadsheet string=w828:string)
                        n249 = call "MaxEye_ATE_Create Configuration Value Header.vi"("Class_value"=w828, "Label_name"=w835, "Class_name"=w836) -> ("Encoded Value"=w827:string)  [unwired: 8 in]
                      }
                      frame "I64" {
                        n250 = Variant To Data(error in=w845, type=i64[][][] [], Variant=w844) -> (data=w842:i64[][][], error out=w837:errorcluster)
                        n251 = Array To Spreadsheet String(delimiter (Tab)=",", array=w842, 3:"%s" ("format string")) -> (spreadsheet string=w839:string)
                        n252 = call "MaxEye_ATE_Create Configuration Value Header.vi"("Class_value"=w839, "Label_name"=w846, "Class_name"=w847) -> ("Encoded Value"=w838:string)  [unwired: 8 in]
                      }
                      frame "U8" {
                        n253 = Variant To Data(error in=w856, type=u8[][][] [], Variant=w855) -> (data=w853:u8[][][], error out=w848:errorcluster)
                        n254 = Array To Spreadsheet String(delimiter (Tab)=",", array=w853, 3:"%s" ("format string")) -> (spreadsheet string=w850:string)
                        n255 = call "MaxEye_ATE_Create Configuration Value Header.vi"("Class_value"=w850, "Label_name"=w857, "Class_name"=w858) -> ("Encoded Value"=w849:string)  [unwired: 8 in]
                      }
                      frame "U16" {
                        n256 = Variant To Data(error in=w867, type=u16[][][] [], Variant=w866) -> (data=w864:u16[][][], error out=w859:errorcluster)
                        n257 = Array To Spreadsheet String(delimiter (Tab)=",", array=w864, 3:"%s" ("format string")) -> (spreadsheet string=w861:string)
                        n258 = call "MaxEye_ATE_Create Configuration Value Header.vi"("Class_value"=w861, "Label_name"=w868, "Class_name"=w869) -> ("Encoded Value"=w860:string)  [unwired: 8 in]
                      }
                      frame "U32" {
                        n259 = Variant To Data(error in=w878, type=u32[][][] [], Variant=w877) -> (data=w875:u32[][][], error out=w870:errorcluster)
                        n260 = Array To Spreadsheet String(delimiter (Tab)=",", array=w875, 3:"%s" ("format string")) -> (spreadsheet string=w872:string)
                        n261 = call "MaxEye_ATE_Create Configuration Value Header.vi"("Class_value"=w872, "Label_name"=w879, "Class_name"=w880) -> ("Encoded Value"=w871:string)  [unwired: 8 in]
                      }
                      frame "U64" {
                        n262 = Variant To Data(error in=w889, type=u64[][][] [], Variant=w888) -> (data=w886:u64[][][], error out=w881:errorcluster)
                        n263 = Array To Spreadsheet String(delimiter (Tab)=",", array=w886, 3:"%s" ("format string")) -> (spreadsheet string=w883:string)
                        n264 = call "MaxEye_ATE_Create Configuration Value Header.vi"("Class_value"=w883, "Label_name"=w890, "Class_name"=w891) -> ("Encoded Value"=w882:string)  [unwired: 8 in]
                      }
                      frame "Single Float" {
                        n265 = Variant To Data(error in=w900, type=sgl[][][] [], Variant=w899) -> (data=w897:sgl[][][], error out=w892:errorcluster)
                        n266 = Array To Spreadsheet String(delimiter (Tab)=",", array=w897, 3:"%s" ("format string")) -> (spreadsheet string=w894:string)
                        n267 = call "MaxEye_ATE_Create Configuration Value Header.vi"("Class_value"=w894, "Label_name"=w901, "Class_name"=w902) -> ("Encoded Value"=w893:string)  [unwired: 8 in]
                      }
                      frame "Double Float" {
                        n268 = Variant To Data(error in=w911, type=dbl[][][] [], Variant=w910) -> (data=w908:dbl[][][], error out=w903:errorcluster)
                        n269 = Array To Spreadsheet String(delimiter (Tab)=",", array=w908, 3:"%s" ("format string")) -> (spreadsheet string=w905:string)
                        n270 = call "MaxEye_ATE_Create Configuration Value Header.vi"("Class_value"=w905, "Label_name"=w912, "Class_name"=w913) -> ("Encoded Value"=w904:string)  [unwired: 8 in]
                      }
                      frame "Extended Float" {
                        n271 = Variant To Data(error in=w922, type=ext[][][] [], Variant=w921) -> (data=w919:ext[][][], error out=w914:errorcluster)
                        n272 = Array To Spreadsheet String(delimiter (Tab)=",", array=w919, 3:"%s" ("format string")) -> (spreadsheet string=w916:string)
                        n273 = call "MaxEye_ATE_Create Configuration Value Header.vi"("Class_value"=w916, "Label_name"=w923, "Class_name"=w924) -> ("Encoded Value"=w915:string)  [unwired: 8 in]
                      }
                      frame "Single Complex" {
                        n274 = Variant To Data(error in=w933, type=ext[][][] [], Variant=w932) -> (data=w930:ext[][][], error out=w925:errorcluster)
                        n275 = Array To Spreadsheet String(delimiter (Tab)=",", array=w930, 3:"%s" ("format string")) -> (spreadsheet string=w927:string)
                        n276 = call "MaxEye_ATE_Create Configuration Value Header.vi"("Class_value"=w927, "Label_name"=w934, "Class_name"=w935) -> ("Encoded Value"=w926:string)  [unwired: 8 in]
                      }
                      frame "Double Complex" {
                        n277 = Variant To Data(error in=w944, type=ext[][][] [], Variant=w943) -> (data=w941:ext[][][], error out=w936:errorcluster)
                        n278 = Array To Spreadsheet String(delimiter (Tab)=",", array=w941, 3:"%s" ("format string")) -> (spreadsheet string=w938:string)
                        n279 = call "MaxEye_ATE_Create Configuration Value Header.vi"("Class_value"=w938, "Label_name"=w945, "Class_name"=w946) -> ("Encoded Value"=w937:string)  [unwired: 8 in]
                      }
                      frame "Extended Complex" {
                        n280 = Variant To Data(error in=w955, type=ext[][][] [], Variant=w954) -> (data=w952:ext[][][], error out=w947:errorcluster)
                        n281 = Array To Spreadsheet String(delimiter (Tab)=",", array=w952, 3:"%s" ("format string")) -> (spreadsheet string=w949:string)
                        n282 = call "MaxEye_ATE_Create Configuration Value Header.vi"("Class_value"=w949, "Label_name"=w956, "Class_name"=w957) -> ("Encoded Value"=w948:string)  [unwired: 8 in]
                      }
                      frame "Enum U8" {
                        n283 = Variant To Data(error in=w966, type=u8[][][] [], Variant=w965) -> (data=w963:u8[][][], error out=w958:errorcluster)
                        n284 = Array To Spreadsheet String(delimiter (Tab)=",", array=w963, 3:"%s" ("format string")) -> (spreadsheet string=w960:string)
                        n285 = call "MaxEye_ATE_Create Configuration Value Header.vi"("Class_value"=w960, "Label_name"=w967, "Class_name"=w968) -> ("Encoded Value"=w959:string)  [unwired: 8 in]
                      }
                      frame "Enum U16" {
                        n286 = Variant To Data(error in=w977, type=u16[][] [], Variant=w976) -> (data=w974:u16[][], error out=w969:errorcluster)
                        n287 = Array To Spreadsheet String(delimiter (Tab)=",", array=w974, 3:"%s" ("format string")) -> (spreadsheet string=w971:string)
                        n288 = call "MaxEye_ATE_Create Configuration Value Header.vi"("Class_value"=w971, "Label_name"=w978, "Class_name"=w979) -> ("Encoded Value"=w970:string)  [unwired: 8 in]
                      }
                      frame "Enum U32" {
                        n289 = Variant To Data(error in=w988, type=u32[][][] [], Variant=w987) -> (data=w985:u32[][][], error out=w980:errorcluster)
                        n290 = Array To Spreadsheet String(delimiter (Tab)=",", array=w985, 3:"%s" ("format string")) -> (spreadsheet string=w982:string)
                        n291 = call "MaxEye_ATE_Create Configuration Value Header.vi"("Class_value"=w982, "Label_name"=w989, "Class_name"=w990) -> ("Encoded Value"=w981:string)  [unwired: 8 in]
                      }
                      frame "Enum U64" {
                        n292 = Variant To Data(error in=w999, type=u64[][][] [], Variant=w998) -> (data=w996:u64[][][], error out=w991:errorcluster)
                        n293 = Array To Spreadsheet String(delimiter (Tab)=",", array=w996, 3:"%s" ("format string")) -> (spreadsheet string=w993:string)
                        n294 = call "MaxEye_ATE_Create Configuration Value Header.vi"("Class_value"=w993, "Label_name"=w1000, "Class_name"=w1001) -> ("Encoded Value"=w992:string)  [unwired: 8 in]
                      }
                      frame "String" {
                        n295 = Variant To Data(error in=w1010, type=string[][][] [], Variant=w1009) -> (data=w1007:string[][][], error out=w1002:errorcluster)
                        n296 = Array To Spreadsheet String(delimiter (Tab)=",", array=w1007, 3:"%s" ("format string")) -> (spreadsheet string=w1004:string)
                        n297 = call "MaxEye_ATE_Create Configuration Value Header.vi"("Class_value"=w1004, "Label_name"=w1011, "Class_name"=w1012) -> ("Encoded Value"=w1003:string)  [unwired: 8 in]
                      }
                      frame "Boolean" {
                        n298 = Variant To Data(error in=w1022, type=bool[][][] [], Variant=w1021) -> (data=w1019:bool[][][], error out=w1013:errorcluster)
                        n299 = Boolean To (0,1)(Boolean=w1019) -> (0, 1=w1014:i16[][][])
                        n300 = Array To Spreadsheet String(delimiter (Tab)=",", array=w1014, 3:"%s" ("format string")) -> (spreadsheet string=w1016:string)
                        n301 = call "MaxEye_ATE_Create Configuration Value Header.vi"("Class_value"=w1016, "Label_name"=w1023, "Class_name"=w1024) -> ("Encoded Value"=w1015:string)  [unwired: 8 in]
                      }
                      frame "Void", Default {
                      }
                    }
                  }
                }
              }
            }
            n302 = Concatenate Strings(w276, w269) -> (w275:string)
          }
          frame "Cluster" {
            n303 = call "MaxEye_ATE_UDS_Create Configuration Variable to Text.vi"("Variant"=w1026, "error in (no error)"=w1031) -> ("concatenated string"=w1027:string, "error out"=w1028:errorcluster)  [unwired: 12 in]
            n304 = Concatenate Strings(w1030, w1027) -> (w1029:string)
          }
        }
      }
      n305 = Concatenate Strings(w20, w18, w19) -> (w17:string)
    }
    frame Error {
    }
  }
  "concatenated string" <- w4
  "error out" <- w2
